vi "1D Inverse DST.vi"(11 "DST {X}":dbl[](array[numeric])) -> (0 "error":i32, 3 "X":dbl[](array[numeric]))   [LabVIEW 2020, in "NI_AALPro.lvlib"]
doc: "Computes the inverse Discrete Sine Transform (DST) of the input sequence <B>DST {X}</B>. Wire data to the <B>DST {X}</B> input to determine the polymorphic instance to use or manually select the instance."
uses:
  NI_AALPro.lvlib
  <resource>/lvanlys.dll
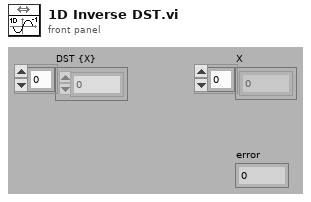
[diagram p1: front panel]
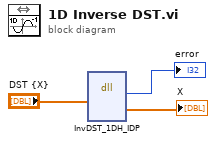
[diagram p0: block diagram]
diagram:
  n1 = dll-call lib="C:/Program Files (x86)/National Instruments/LabVIEW 2020/resource/lvanlys.*" fn="InvDST_1DH_IDP"("xH"="DST {X}") -> ("return type"=→"error":i32, "yH"=→"X":dbl[])  [unwired: 7 in, 2 out]
